vi "qcpTest.vi"() -> ()   [LabVIEW 2017]
uses:
  <userlib>/836-Library/System/QCP_V2/QCPSupportCode/QCP_GetDbl.vi
  <userlib>/836-Library/System/QCP_V2/QCPSupportCode/QCP_GetDblArr.vi
  <userlib>/836-Library/System/QCP_V2/QCPSupportCode/QCP_SetDblArr.vi
  <userlib>/836-Library/System/QCP_V2/QCPSupportCode/QCP_SetDbl.vi
  <userlib>/836-Library/System/QCP_V2/QCPSupportCode/QCPData.ctl
panel:
  out "three":dbl[](array[numeric])
  out "one":dbl
  out "thirty":dbl[](array[numeric])
  out "ten":dbl
  out "data value":T1
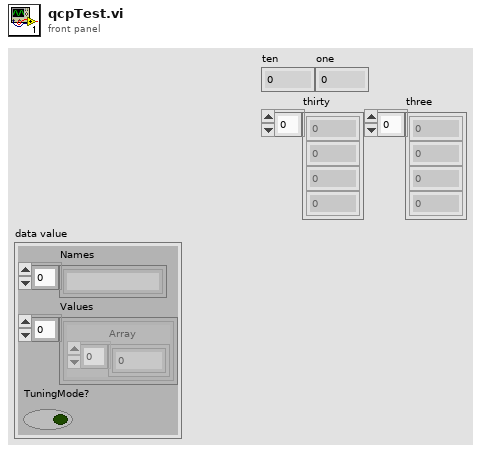
[diagram p1: front panel]
types:
  T1 = typedef "QCPData.ctl" = cluster{"Names":string[], "Values":cluster{"Array":dbl[]}[], "TuningMode?":bool}
  T2 = typedef "QCP_RefNum.ctl" = cluster{"Data Value Refnum":refnum<data-value>, "semaphore":T3}
  T3 = typedef "Semaphore RefNum" = refnum<k1>
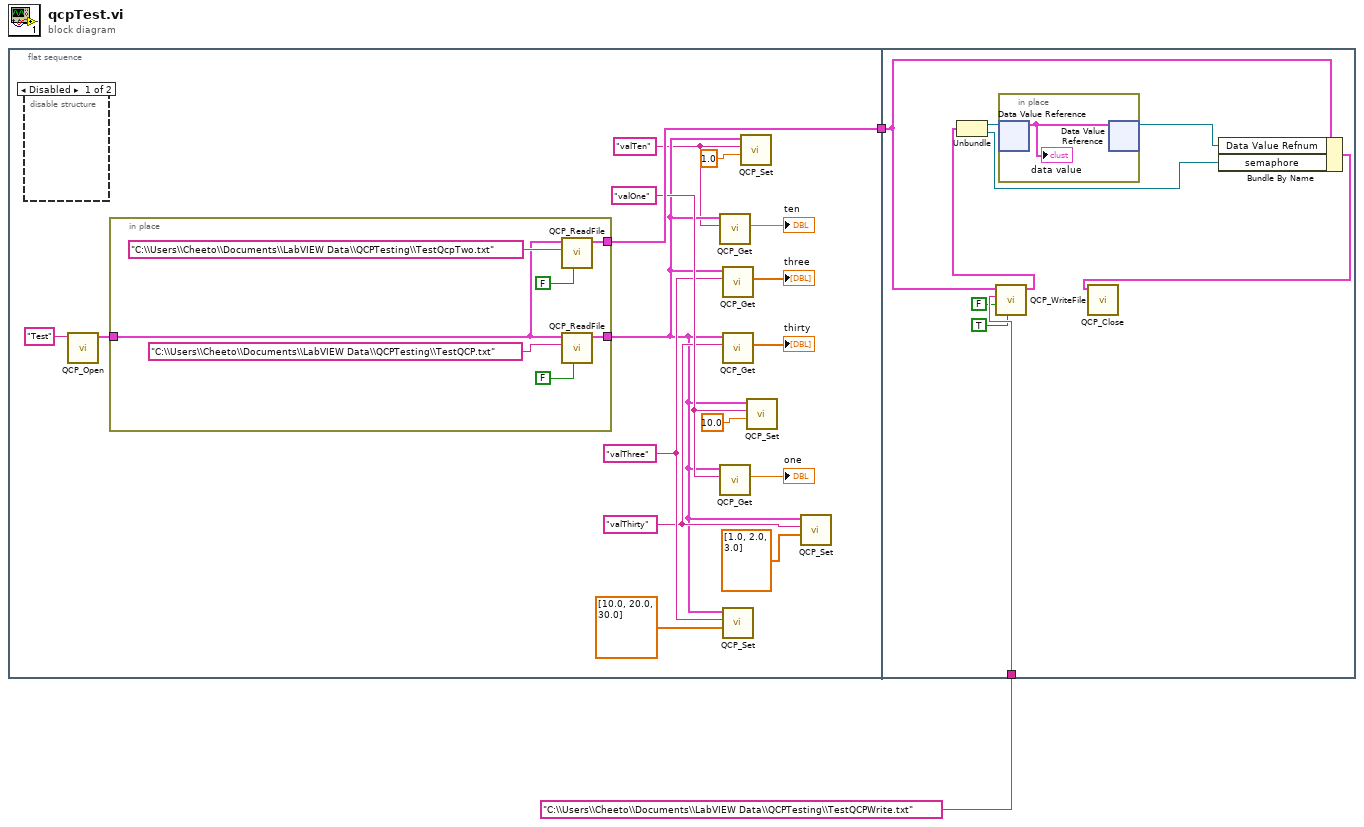
[diagram p0: block diagram]
diagram:
  n1 = flat-sequence {
    tunnel: [w17] -> w2
    tunnel: w2 -> [w30]
    tunnel: "C:\\Users\\Cheeto\\Documents\\LabVIEW Data\\QCPTesting\\TestQCPWrite.txt" ("Path") -> [w33]
    frame #0 {
      w9 = "valThirty" ("Value Name")
      w7 = "valTen" ("Value Name")
      w10 = "valThree" ("Value Name")
      w11 = "valOne" ("Value Name")
      n2 = disable-structure shown="Disabled" {
        frame Disabled {
        }
        frame Enabled {
        }
      }
      n3 = call <userlib>:"QCP_Open.vi"("Name"="Test") -> ("QCP_DevRef_Out"=w16:T2)  [unwired: 9 in, 1 out]
      n4 = in-place {
        in-place-border: [w21] -> w17
        in-place-border: w16 -> [w20]
        in-place-border: [w19] -> w8
        n5 = call <userlib>:"QCP_ReadFile.vi"("Overrite Existing Data?"=FALSE, "Path"="C:\\Users\\Cheeto\\Documents\\LabVIEW Data\\QCPTesting\\TestQcpTwo.txt", "QCP_DevRef_In"=w20) -> ("QCP_DevRef_Out"=w21:T2)  [unwired: 7 in, 1 out]
        n6 = call <userlib>:"QCP_ReadFile.vi"("Overrite Existing Data?"=FALSE, "Path"="C:\\Users\\Cheeto\\Documents\\LabVIEW Data\\QCPTesting\\TestQCP.txt", "QCP_DevRef_In"=w20) -> ("QCP_DevRef_Out"=w19:T2)  [unwired: 7 in, 1 out]
      }
      n7 = call-poly <userlib>:"QCP_Get.vi"("Value Name"=w7, "QCP_DevRef_In"=w8) -> ("Value"=→"ten":dbl)  [unwired: 7 in, 2 out]
      n8 = call-poly <userlib>:"QCP_Get.vi"("Value Name"=w11, "QCP_DevRef_In"=w8) -> ("Value"=→"one":dbl)  [unwired: 7 in, 2 out]
      n9 = call-poly <userlib>:"QCP_Get.vi"("Value Name"=w10, "QCP_DevRef_In"=w8) -> ("Values"=→"three":dbl[])  [unwired: 7 in, 2 out]
      n10 = call-poly <userlib>:"QCP_Get.vi"("Value Name"=w9, "QCP_DevRef_In"=w8) -> ("Values"=→"thirty":dbl[])  [unwired: 7 in, 2 out]
      n11 = call-poly <userlib>:"QCP_Set.vi"("Values"=dbl[] [10.0, 20.0, 30.0], "Name"=w10, "QCP_DevRef_In"=w8) -> ()  [unwired: 7 in, 2 out]
      n12 = call-poly <userlib>:"QCP_Set.vi"("Value"=1.0, "Name"=w7, "QCP_DevRef_In"=w8) -> ()  [unwired: 7 in, 2 out]
      n13 = call-poly <userlib>:"QCP_Set.vi"("Value"=10.0, "Name"=w11, "QCP_DevRef_In"=w8) -> ()  [unwired: 7 in, 2 out]
      n14 = call-poly <userlib>:"QCP_Set.vi"("Values"=dbl[] [1.0, 2.0, 3.0], "Name"=w9, "QCP_DevRef_In"=w8) -> ()  [unwired: 7 in, 2 out]
    }
    frame #1 {
      n15 = call <userlib>:"QCP_WriteFile.vi"("Overrite?"=TRUE, "Path relative?"=FALSE, "Path"=w33, "QCP_DevRef_In"=w30) -> ("QCP_DevRef_Out"=w26:T2)  [unwired: 6 in, 1 out]
      n16 = Unbundle(w26) -> ("Data Value Refnum"=w34:refnum<data-value>, "semaphore"=w28:T3)
      n17 = in-place {
        n18 = in-place-dvr #1(w34) -> (w35:T1)  [unwired: 1 out]
        "data value" <- w35
        n19 = in-place-dvr #1(w35) -> (w29:refnum<data-value>)  [unwired: 1 out]
      }
      n20 = Bundle By Name(cluster=w30, "Data Value Refnum"=w29, "semaphore"=w28) -> (w27:T2)
      n21 = call <userlib>:"QCP_Close.vi"("QCP_DevRef_In"=w27) -> ()  [unwired: 10 in, 1 out]
    }
  }
